vi "Create LVClass for Oneof.vi"(7 "Message Elements":T1[](array[typedef]), 8 "error in (no error)":errorcluster, 9 "Message Name":string, 10 "Parent Message Typedef":refnum<vi>, 11 "library in":refnum<vi>) -> (0 "error out":errorcluster, 3 "library out":refnum<vi>)   [LabVIEW 2019, in "gRPC Template Creation Utility.lvlib"]
uses:
  gRPC Template Creation Utility.lvlib
  TypeDefs/Message Element Metadata (Scripting).ctl
  TypeDefs/Message Element Type.ctl
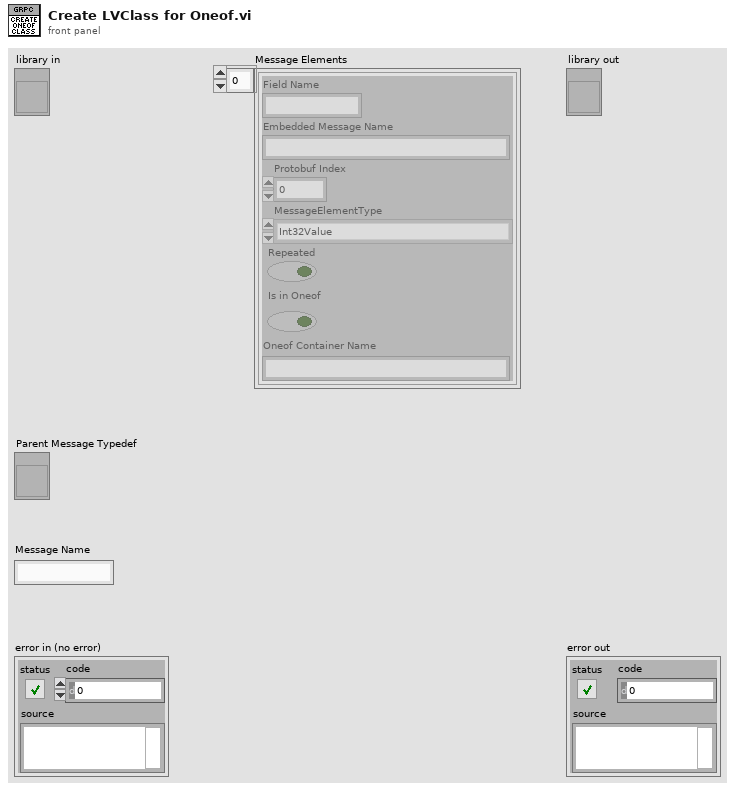
[diagram p1: front panel]
types:
  T1 = typedef "gRPC Template Creation Utility.lvlib/Message Element Metadata (Scripting).ctl" = cluster{"Field Name":string, "Embedded Message Name":string, "Protobuf Index":i32, "MessageElementType":T2, "Repeated":bool, "Is in Oneof":bool, "Oneof Container Name":string}
  T2 = typedef "gRPC Template Creation Utility.lvlib/Message Element Type.ctl" = enum32{"Int32Value", "FloatValue", "DoubleValue", "BoolValue", "StringValue", "MessageValue", "Int64Value", "UInt32Value", "UInt64Value", "EnumValue", "Bytes", "Fixed64", "Fixed32", "SFixed64", "SFixed32", "SInt64", "SInt32"}
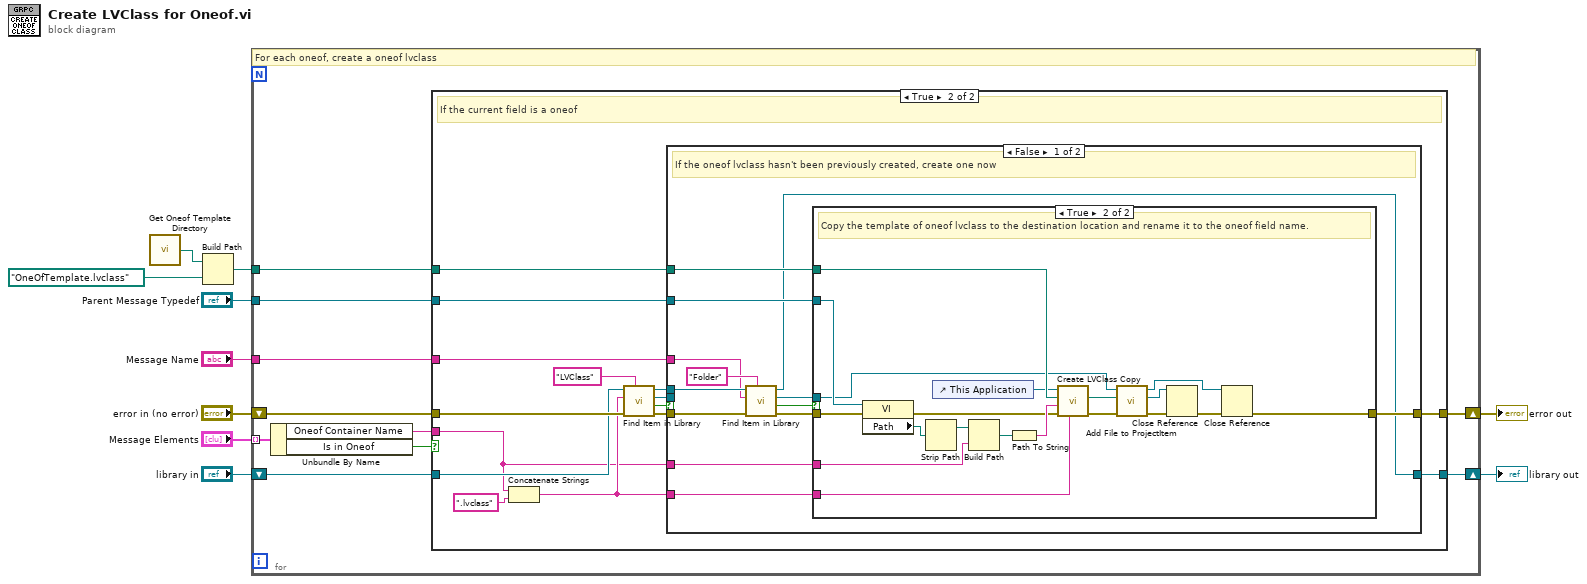
[diagram p0: block diagram]
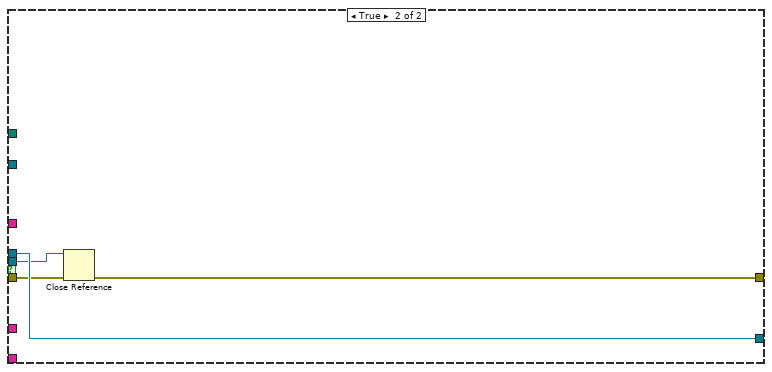
[diagram p4: hidden frame]
diagram:
  n1 = call "Get Oneof Template Directory.vi"() -> ("appended path"=w3:path)
  n2 = Build Path(base path=w3, name or relative path=path "OneOfTemplate.lvclass") -> (appended path=w2:path)
  n3 = for {
    tunnel: "Message Elements" -> [w20] mode=indexing
    tunnel: "Message Name" -> [w16]
    tunnel: "Parent Message Typedef" -> [w13]
    tunnel: w2 -> [w12]
    shift-right: [w17] -> w9
    shift-left: "error in (no error)" -> [w18]
    shift-right: [w14] -> w6
    shift-left: "library in" -> [w15]
    # "For each oneof, create a oneof lvclass"
    n4 = Unbundle By Name(w20) -> ("Oneof Container Name"=w11:string, "Is in Oneof"=w19:bool)
    n5 = case shown="True" w19 {
      tunnel: [w22 w37] -> w17
      tunnel: w18 -> [w22 w34]
      tunnel: w16 -> [_ w36]
      tunnel: w15 -> [w21 w33]
      tunnel: [w21 w35] -> w14
      tunnel: w13 -> [_ w27]
      tunnel: w12 -> [_ w26]
      tunnel: w11 -> [_ w24]
      frame False {
      }
      frame True {
        # "If the current field is a oneof"
        n6 = Concatenate Strings(w24, ".lvclass" ("string")) -> (w25:string)
        n7 = call "Find Item in Library.vi"("Item Type"="LVClass", "error in (no error)"=w34, "Item Name"=w25, "Library item in"=w33) -> ("error out"=w29:errorcluster, "Found?"=w28:bool, "Project Item (Library Item)"=w23:refnum<vi>, "Library item out"=w32:refnum<vi>)  [unwired: 4 in]
        n8 = case shown="False" w28 {
          tunnel: [w46 w72] -> w37
          tunnel: w24 -> [w45 _]
          tunnel: w36 -> [w42 _]
          tunnel: [w38 w74] -> w35
          tunnel: w32 -> [w43 w74]
          tunnel: w29 -> [w44 w73]
          tunnel: w27 -> [w41 _]
          tunnel: w26 -> [w40 _]
          tunnel: w25 -> [w39 _]
          tunnel: w23 -> [_ w71]
          frame False {
            # "If the oneof lvclass hasn't been previously created, create one now"
            n9 = call "Find Item in Library.vi"("Item Type"="Folder", "error in (no error)"=w44, "Item Name"=w42, "Library item in"=w43) -> ("error out"=w48:errorcluster, "Found?"=w47:bool, "Project Item (Library Item)"=w50:refnum<vi>, "Library item out"=w38:refnum<vi>)  [unwired: 4 in]
            n10 = case shown="True" w47 {
              tunnel: w45 -> [_ w58]
              tunnel: w50 -> [_ w55]
              tunnel: [w51 w53] -> w46
              tunnel: w48 -> [w51 w64]
              tunnel: w41 -> [_ w68]
              tunnel: w40 -> [_ w66]
              tunnel: w39 -> [_ w57]
              frame False {
                # "Container message should have been created already."
              }
              frame True {
                # "Copy the template of oneof lvclass to the destination location and rename it to the oneof field name."
                n11 = property class="VI"(reference=w68, error in=w64) -> (error out=w63:errorcluster, "Path"=w69:path)  [unwired: 1 out]
                n12 = Strip Path(path=w69) -> (stripped path=w60:path)  [unwired: 1 out]
                n13 = control-ref of="This Application"() -> (w61:refnum<vi>)
                n14 = Build Path(base path=w60, name or relative path=w58) -> (appended path=w59:path)
                n15 = Path To String(path=w59) -> (string=w65:string)
                n16 = call "Create LVClass Copy.vi"("New Name"=w57, "error in (no error)"=w63, "New Path"=w65, "Source Class Path"=w66, "Application in"=w61) -> ("error out"=w62:errorcluster, "Copy Class Path out"=w56:path)  [unwired: 4 in, 1 out]
                n17 = call "Add File to ProjectItem.vi"("error in (no error)"=w62, "File Path"=w56, "ProjectItem in"=w55) -> ("error out"=w67:errorcluster, "Added File ref"=w70:refnum<vi>, "ProjectItem out"=w52:refnum<vi>)  [unwired: 6 in]
                n18 = Close Reference(reference=w70, error in (no error)=w67) -> (error out=w54:errorcluster)
                n19 = Close Reference(reference=w52, error in (no error)=w54) -> (error out=w53:errorcluster)
              }
            }
          }
          frame True {
            n20 = Close Reference(reference=w71, error in (no error)=w73) -> (error out=w72:errorcluster)
          }
        }
      }
    }
  }
  "error out" <- w9
  "library out" <- w6
